vi "Manual EMS.vi"(8 "error in":errorcluster, 11 "Master Controller in":refnum<class "EMS User Interface.lvclass">) -> (0 "error out":errorcluster, 3 "dup Master Controller out":refnum<class "EMS User Interface.lvclass">)   [LabVIEW 2018, in "EMS User Interface Actor.lvlib" / "EMS User Interface.lvclass"]
uses:
  EMS User Interface.lvclass
  EMS User Interface.lvclass/EMS User Interface.ctl
  EMS Core/EMS/Controls/Microgrid State.ctl
  <vilib>/ActorFramework/Message Enqueuer/Message Priority.ctl
  <vilib>/ActorFramework/Message Enqueuer/Message Enqueuer.lvclass/Message Enqueuer.ctl
  <vilib>/ActorFramework/Message Enqueuer/Enqueue.vi
  EMS Core/EMS Messages/Stop Init Msg/Stop Init Msg.lvclass
  C:/Program Files (x86)/National Instruments/LabVIEW 2018/vi.lib/ActorFramework/Message/Message.lvclass
  <vilib>/ActorFramework/Message Priority Queue/Priority Enqueue.vi
  <vilib>/ActorFramework/Message Enqueuer/Message Enqueuer.lvclass
  EMS Core/EMS/EMS.lvclass
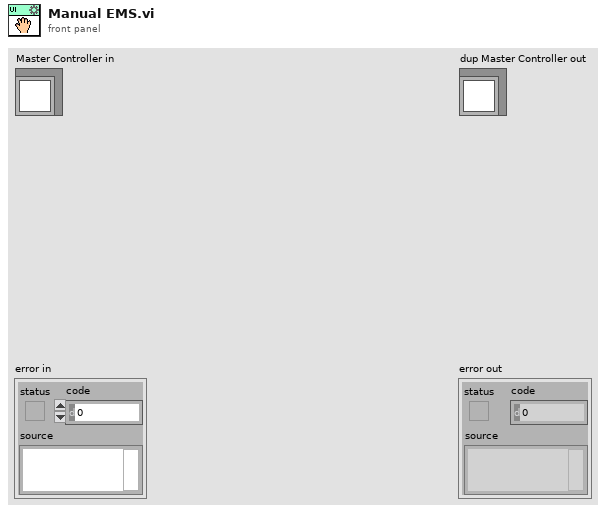
[diagram p1: front panel]
types:
  T1 = typedef "Actor Framework.lvlib/Message Enqueuer.lvclass/Message Priority.ctl" = enum16{"Low", "Normal", "High"}
  T2 = typedef "EMS Core.lvlib/EMS.lvclass/Microgrid State.ctl" = enum16{"Discovery", "Commissioning", "Activation", "Blackstart", "OnGrid", "OffGrid", "Island", "Resynchronization", "Manual", "Shutdown", "Stop"}
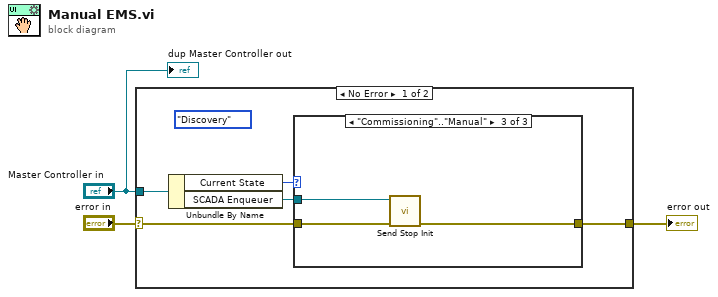
[diagram p0: block diagram]
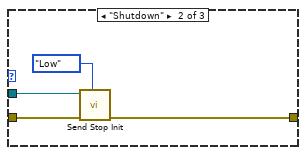
[diagram p3: hidden frame]
diagram:
  n1 = case shown="No Error" "error in" {
    selector: "error in" -> [w7 w17]
    tunnel: [w8 w17] -> w2
    tunnel: "Master Controller in" -> [w5 _]
    frame No Error {
      (unwired) Microgrid_State."Discovery" ("Current State")
      n2 = Unbundle By Name(w5) -> ("Current State"=w6:T2, "SCADA Enqueuer"=w4:refnum<class "Message Enqueuer.lvclass">)
      n3 = case shown="\"Commissioning\"..\"Manual\"" w6 {
        tunnel: [w9 w12 w14] -> w8
        tunnel: w7 -> [w9 w13 w15]
        tunnel: w4 -> [_ w11 w16]
        frame "Discovery", Default {
        }
        frame "Shutdown" {
          n4 = call "Send Stop Init.vi"("Message Priority (Normal)"=Message_Priority."Low", "error in (no error)"=w13, "Message Enqueuer"=w11) -> ("error out"=w12:errorcluster)  [unwired: 7 in, 1 out]
        }
        frame "Commissioning".."Manual" {
          n5 = call "Send Stop Init.vi"("error in (no error)"=w15, "Message Enqueuer"=w16) -> ("error out"=w14:errorcluster)  [unwired: 8 in, 1 out]
        }
      }
    }
    frame Error {
    }
  }
  "error out" <- w2
  "dup Master Controller out" <- "Master Controller in"
